vi "Weather Station UI_EX.vi"() -> ()   [LabVIEW 2021]
doc: "This is the main VI in the Weather Station project. It contains the user interface for a temperature warning system. Temperature is retrieved every half second; data is logged when a warning has occurred."
uses:
  Instance           2 26Saved   Weather Station UI .vi
panel:
  out "Warning":string
  in  "Lower Limit":dbl=20.0
  in  "Upper Limit":dbl=30.0
  in  "Stop Button":bool
  out "Temperature History":dbl(graph)
  # "Temperature Ranges (C)"
  # "Freeze"
  # "Heat \nStroke"
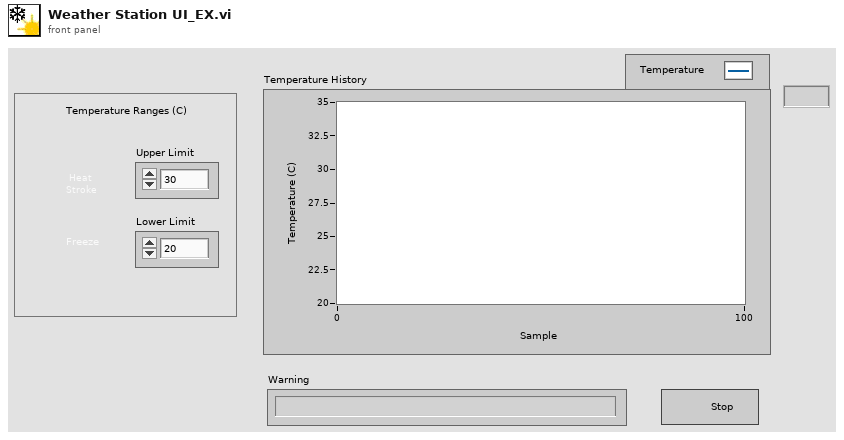
[diagram p1: front panel]
types:
  T1 = enum16{"open", "replace", "create", "open or create", "replace or create", "replace or create with confirmation"}
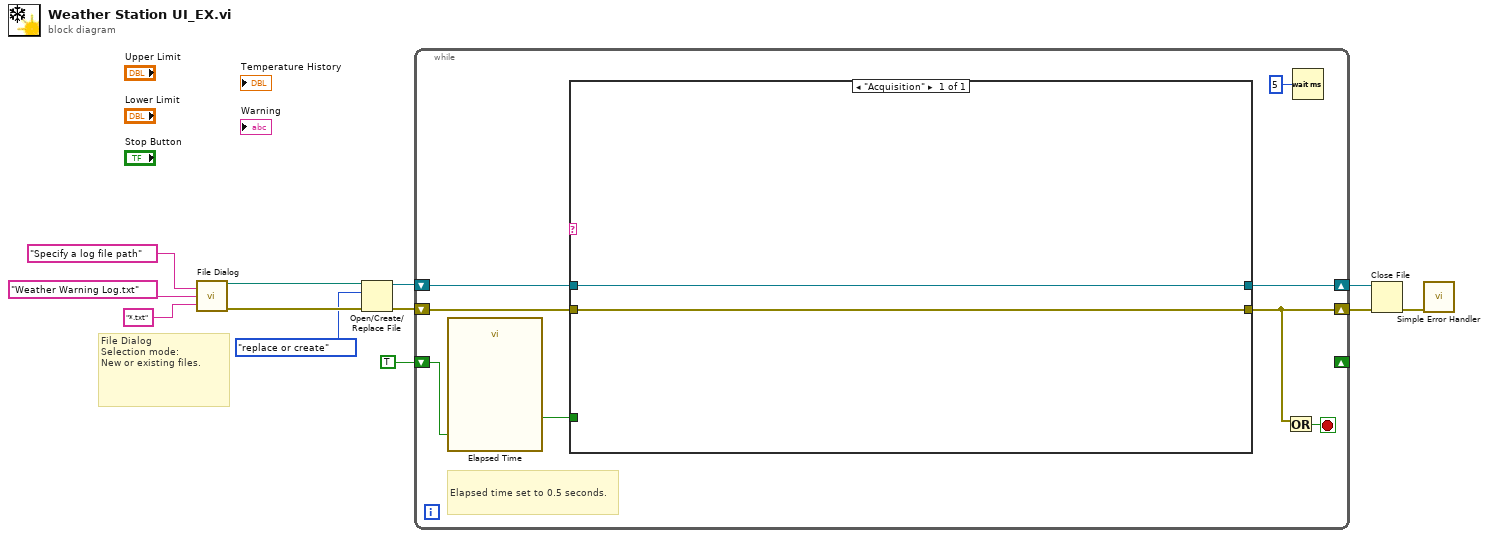
[diagram p0: block diagram]
diagram:
  # "File Dialog\nSelection mode:\nNew or existing files."
  n1 = call "File Dialog"("prompt"="Specify a log file path", "default name"="Weather Warning Log.txt", "pattern (all files)"="*.txt" ("pattern label")) -> ("selected path"=w6:path, "error out"=w3:errorcluster)  [unwired: 9 in, 2 out]
  n2 = Open/Create/Replace File(file path (use dialog)=w6, error in=w3, operation (0:open)=T1."replace or create") -> (refnum out=w8:refnum<file>, error out=w7:errorcluster)  [unwired: 3 in, 1 out]
  n3 = while {
    shift-right: [w13] -> w12
    shift-left: w7 -> [w20]
    shift-right: [w18] -> w11
    shift-left: w8 -> [w17]
    shift-right: _ -> [_]
    shift-left: TRUE ("stop") -> [w15]
    stop <- w19 stop-if-true
    # "Elapsed time set to 0.5 seconds."
    n4 = call "Elapsed Time"("Reset"=w15) -> ("Time has Elapsed"=w14:bool)  [unwired: 11 in, 7 out]
    n5 = case shown="\"Acquisition\"" {
      selector: _ -> [_]
      tunnel: [w21] -> w13
      tunnel: w20 -> [w21]
      tunnel: [w22] -> w18
      tunnel: w17 -> [w22]
      tunnel: w14 -> [_]
      frame "Acquisition" {
      }
    }
    n6 = Or(x=w13) -> (x .or. y?=w19:bool)  [unwired: 1 in]
    n7 = Wait (ms)(milliseconds to wait=u32 5 ("y")) -> ()  [unwired: 1 out]
  }
  n8 = Close File(refnum=w11, error in=w12) -> (error out=w10:errorcluster)  [unwired: 1 out]
  n9 = call <vilib>:"Simple Error Handler.vi"("error in (no error)"=w10) -> ()  [unwired: 4 in, 5 out]
